vi "AMWave.vi"() -> ()   [LabVIEW 2015]
uses:
  <vilib>/imath/engines/lvmath2/RunTimeEngine/Managers/WorkSpace/UID Generator.vi
  <vilib>/imath/engines/lvmath2/RunTimeEngine/RunTimeType/NIMS_RunTimeType_From StrictType (excl LVString).vi
  <instcachedir>/0/NIMS_RunTimeType_From StrictType (excl LVString)_EB1C38A9BC5048DA9ABDA8F781E54D21.lvgen/NIMS_RunTimeType_From StrictType (excl LVString)_EB1C38A9BC5048DA9ABDA8F781E54D21_000.vi
  <vilib>/imath/engines/lvmath2/RunTimeEngine/LocalVariableDefStatement/MC_LocalVariableDefStatement_Display.vi
  <vilib>/imath/engines/lvmath2/RunTimeEngine/RangeToken/NIMS_Range.vi
  <instcachedir>/0/NIMS_Range_D919CC09935940E88F755EC1C6F49AC1.lvgen/NIMS_Range_D919CC09935940E88F755EC1C6F49AC1_000.vi
  <vilib>/imathl/engines/lvmath/Functions/Error Handling/Create Error.vi
  <vilib>/imath/engines/lvmath2/RunTimeEngine/ArithmeticOperatorToken/NIMS_ArithmeticOperator_multmx.vi
  <instcachedir>/0/NIMS_ArithmeticOperator_multmx_E413577642394AA3A74EB19F669417B0.lvgen/NIMS_ArithmeticOperator_multmx_E413577642394AA3A74EB19F669417B0_004.vi
  <vilib>/imath/engines/lvmath2/RunTimeEngine/NodeEndStatement/NIMS_NodeEndStatement_Get Vector.vi
  <instcachedir>/0/NIMS_NodeEndStatement_Get Vector_ED7FC4F6B50246F79D573C75B2E51AF8.lvgen/NIMS_NodeEndStatement_Get Vector_ED7FC4F6B50246F79D573C75B2E51AF8_001.vi
  <vilib>/imath/engines/lvmath/Functions/Error Handling/MergeErrorsWrapper.vi
  <vilib>/imath/engines/lvmath2/RunTimeEngine/Managers/SymbolTable/Clear UID.vi
  <vilib>/imath/engines/lvmath2/RunTimeEngine/NodeEndStatement/NIMS_NodeEndStatement_Output.vi
  <instcachedir>/0/NIMS_NodeEndStatement_Output_53EC0D466D134D7ABD903AC30B43404B.lvgen/NIMS_NodeEndStatement_Output_53EC0D466D134D7ABD903AC30B43404B_005.vi
  <vilib>/imath/engines/lvmath2/RunTimeEngine/ErrorHandling/NIMS_Finalize Error.vi
  <vilib>/imath/engines/lvmath2/RunTimeEngine/Managers/SymbolTable/NIMS_WorkSpace.lvlib
panel:
  in  "Amplitude":dbl
  in  "Modulation Frequency":dbl
  in  "Signal Frequency":dbl
  out "XY Graph":cluster{"x":dbl[], "t":dbl[]}(graph)
  in  "Sampling Frequency":dbl
  in  "Number of Samples":dbl
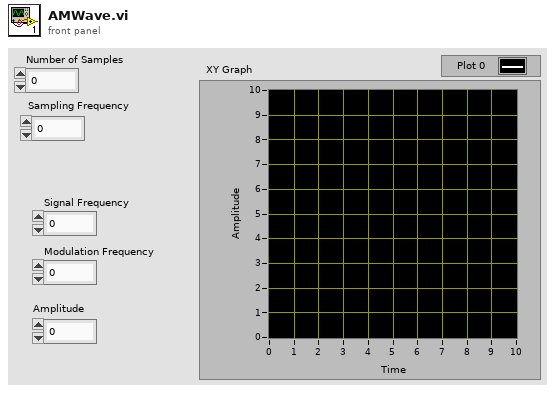
[diagram p1: front panel]
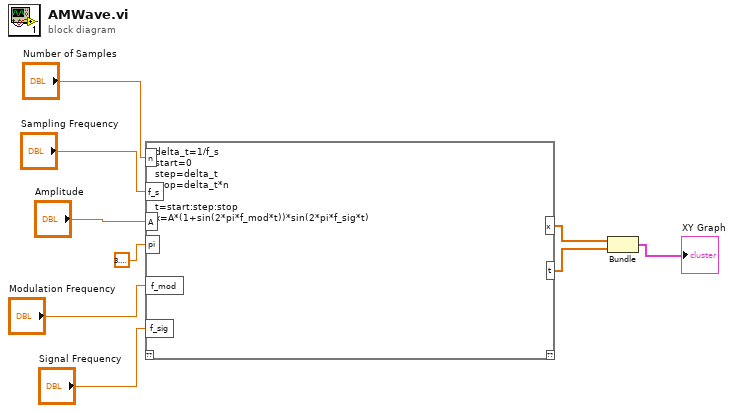
[diagram p0: block diagram]
diagram:
  n1 = mathscript code="delta_t=1/f_s\nstart=0\nstep=delta_t\nstop=delta_t*n\n\nt=start:step:stop\nx=A*(1+sin(2*pi*f_mod*t))*sin(2*pi*f_sig*t)"("pi"=3.141592653589793, "f_mod"="Modulation Frequency", "f_sig"="Signal Frequency", "A"="Amplitude", "f_s"="Sampling Frequency", "n"="Number of Samples") -> ("x"=w3:dbl[], "t"=w2:dbl[])  [unwired: 1 in, 1 out]
  n2 = Bundle("x"=w3, "t"=w2) -> (→"XY Graph":cluster{"x":dbl[], "t":dbl[]})  [unwired: 1 in]
